vi "liftPID.vi"(9 "constantProportion":dbl, 10 "currentValue":dbl, 11 "setValue":dbl) -> (3 "motorOutput":dbl)   [LabVIEW 2014]
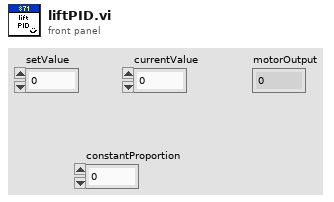
[diagram p1: front panel]
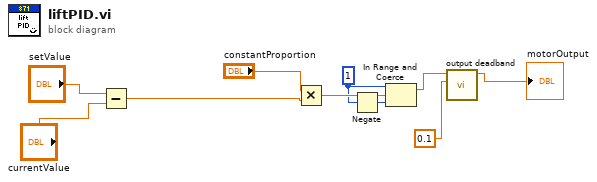
[diagram p0: block diagram]
diagram:
  w4 = 1
  n1 = Subtract(x="setValue", y="currentValue") -> (x-y=w7:dbl)
  n2 = Multiply(x="constantProportion", y=w7) -> (x*y=w6:dbl)
  n3 = Negate(x=w4) -> (-x=w5:i32)
  n4 = In Range and Coerce(upper limit=w4, x=w6, lower limit=w5) -> (coerced(x)=w1:dbl)  [unwired: 1 out]
  n5 = call "output deadband.vi"("deadband width"=0.1, "motor input"=w1) -> ("motor output"=→"motorOutput":dbl)  [unwired: 9 in]
